vi "session_check_list.vi"(7 "VISA resource names in":refnum<visa-resource-name>[](array[refnum]), 8 "error in":errorcluster, 10 "Error if not found (T)":bool=TRUE, 11 "VISA resource name":refnum<visa-resource-name>) -> (0 "error out":errorcluster, 2 "Found in the list":bool, 3 "Session list index out":i32)   [LabVIEW 2014, in "rszvl_rsidr_core.lvlib"]
uses:
  rszvl_rsidr_core.lvlib
  type_Error_Codes.ctl
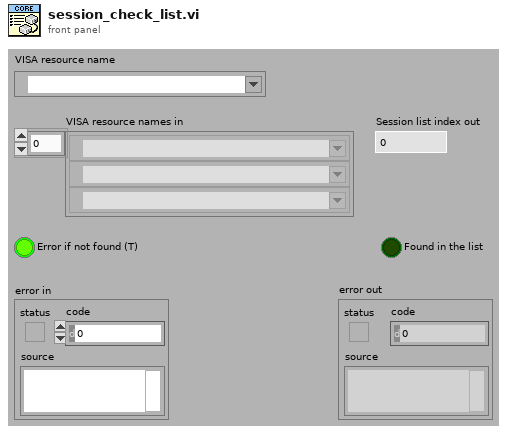
[diagram p1: front panel]
types:
  T1 = typedef "rszvl_rsidr_core.lvlib/type_Error_Codes.ctl" = enum16{"No_error", "VISA_err_ResourceNotFound", "VISA_err_Timeout", "VISA_warn_MoreDataAvailable", "RS_err_MissingCallback", "RS_err_InvalidAttribute", "RS_err_InvalidValue", "RS_err_UnknownResource", "RS_err_AlreadyInitialized", "RS_err_InstrumentStatus", "RS_err_BadRepCapName", "RS_err_TypesMismatch", "RS_err_ValueNotSupported", "RS_err_InvalidRngTable", "RS_err_IDqueryFail", "RS_err_UnexpResponse", "VISA_warn_ConfigNotLoaded", "RS_err_AttributeNotReadable", "RS_err_AttributeNotWritable", "RS_err_InstrumentType", "RS_err_InstrumentOption", "VISA_err_InvalidSize", "RS_err_ReliabilityIndicator", "VISA_warn_UnknownStatus", "VISA_warn_TermCharRead", "VISA_err_IO_error"}
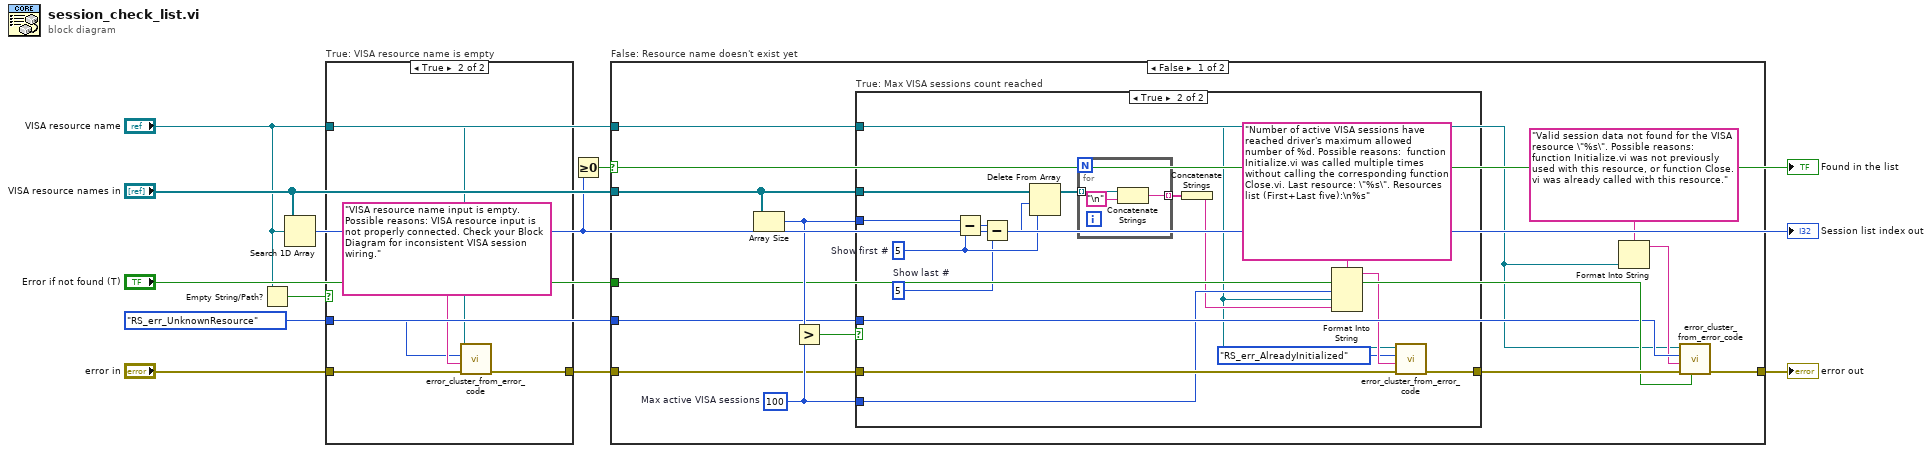
[diagram p0: block diagram]
diagram:
  w2 = type_Error_Codes."RS_err_UnknownResource" ("Error Enum in")
  n1 = Empty String/Path?(string/path="VISA resource name") -> (empty?=w5:bool)
  n2 = Search 1D Array(1D array="VISA resource names in", element="VISA resource name") -> (index of element=w6:i32)  [unwired: 1 in]
  "Session list index out" <- w6
  n3 = case "True: VISA resource name is empty" shown="True" w5 {
    tunnel: "error in" -> [w11 w15]
    tunnel: [w11 w16] -> w4
    tunnel: w2 -> [_ w13]
    tunnel: "VISA resource name" -> [_ w12]
    frame False {
    }
    frame True {
      n4 = call "error_cluster_from_error_code.vi"("error in"=w15, "error message (\"\")"="VISA resource name input is empty. Possible reasons: VISA resource input is not properly connected. Check your Block Diagram for inconsistent VISA session wiring." ("error message (\"\")"), "Error Enum in"=w13, "VISA resource name"=w12) -> ("error out"=w16:errorcluster)  [unwired: 6 in, 1 out]
    }
  }
  n5 = Greater Or Equal To 0?(x=w6) -> (x >= 0?=w8:bool)
  "Found in the list" <- w8
  n6 = case "False: Resource name doesn't exist yet" shown="False" w8 {
    tunnel: w4 -> [w20 w49]
    tunnel: [w23 w49] -> w10
    tunnel: "Error if not found (T)" -> [w22 _]
    tunnel: "VISA resource names in" -> [w27 _]
    tunnel: "VISA resource name" -> [w17 _]
    tunnel: w2 -> [w19 _]
    frame False {
      w21 = 100  # Max active VISA sessions
      n7 = Array Size(array=w27) -> (size(s)=w26:i32)
      n8 = Greater?(x=w26, y=w21) -> (0:w28:bool)
      n9 = case "True: Max VISA sessions count reached" shown="True" w28 {
        tunnel: w20 -> [w29 w45]
        tunnel: w19 -> [_ _]
        tunnel: w21 -> [_ w44]
        tunnel: w17 -> [_ w30]
        tunnel: w27 -> [_ w42]
        tunnel: w26 -> [_ w43]
        tunnel: [w29 w33] -> w24
        frame False {
        }
        frame True {
          w39 = 5  # Show last #
          w41 = 5  # Show first #
          n10 = Subtract(x=w43, y=w41) -> (x-y=w40:i32)
          n11 = Subtract(x=w40, y=w39) -> (x-y=w38:i32)
          n12 = Delete From Array(array=w42, length=w38, index=w41) -> (array with subset deleted=w37:refnum<visa-resource-name>[])  [unwired: 1 out]
          n13 = for {
            tunnel: w37 -> [w48] mode=indexing
            tunnel: [w46] -> w35 mode=indexing
            n14 = Concatenate Strings(w48, "\n" ("Line Feed Constant")) -> (w46:string)
          }
          n15 = Concatenate Strings(w35) -> (w34:string)
          n16 = Format Into String(format string="Number of active VISA sessions have reached driver's maximum allowed number of %d. Possible reasons:  function Initialize.vi was called multiple times without calling the corresponding function Close.vi. Last resource: \"%s\". Resources list (First+Last five):\n%s" ("error message (\"\")"), w44, w30, w34) -> (resulting string=w32:string)  [unwired: 2 in, 1 out]
          n17 = call "error_cluster_from_error_code.vi"("error in"=w45, "error message (\"\")"=w32, "Error Enum in"=type_Error_Codes."RS_err_AlreadyInitialized", "VISA resource name"=w30) -> ("error out"=w33:errorcluster)  [unwired: 6 in, 1 out]
        }
      }
      n18 = Format Into String(format string="Valid session data not found for the VISA resource \"%s\". Possible reasons:  function Initialize.vi was not previously used with this resource, or function Close.vi was already called with this resource." ("error message (\"\")"), w17) -> (resulting string=w18:string)  [unwired: 2 in, 1 out]
      n19 = call "error_cluster_from_error_code.vi"("error creation enabled (T)"=w22, "error in"=w24, "error message (\"\")"=w18, "Error Enum in"=w19, "VISA resource name"=w17) -> ("error out"=w23:errorcluster)  [unwired: 5 in, 1 out]
    }
    frame True {
    }
  }
  "error out" <- w10
